vi "Parameter Channel to Strings.vi"(11 "parameter channel definition":T3={"name"="", "default value"=1.0, "unit"="", "parameter definition"={"start index"=0, "size (bits)"=16, "encoding"=enum."BNR", "signed"=TRUE, "multiplier"=1.0, "offset"=0.0}}) -> (3 "parameter channel strings":T1)   [LabVIEW 2020, in "AIM MIL-STD-1553 System Explorer.lvlib" / "Implementation.lvlib" / "Refresh.lvlib"]
uses:
  Refresh.lvlib
  Shared/Parameter Definition.ctl
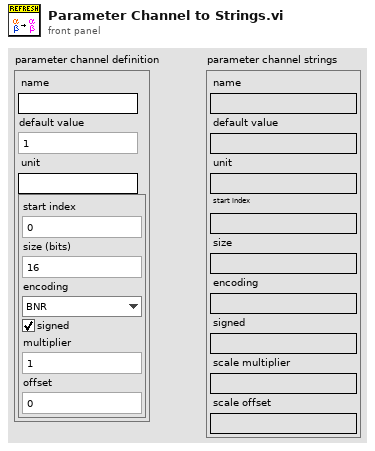
[diagram p1: front panel]
types:
  T1 = cluster{"name":string, "default value":string, "unit":string, "start index":string, "size":string, "encoding":string, "signed":string, "scale multiplier":string, "scale offset":string}
  T2 = typedef "Parameter Definition.ctl" = cluster{"start index":i32, "size (bits)":i32, "encoding":enum16{"BNR", "BCD", "Discrete"}, "signed":bool, "multiplier":dbl, "offset":dbl}
  T3 = cluster{"name":string, "default value":dbl, "unit":string, "parameter definition":T2}
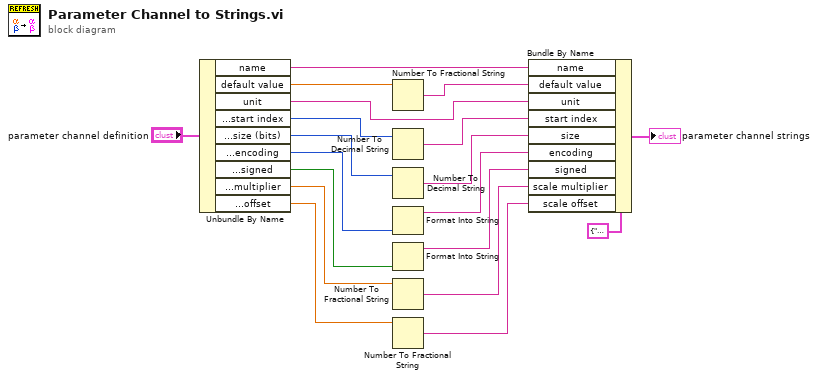
[diagram p0: block diagram]
diagram:
  n1 = Unbundle By Name("parameter channel definition") -> ("name"=w19:string, "default value"=w18:dbl, "unit"=w16:string, "parameter definition.start index"=w15:i32, "parameter definition.size (bits)"=w14:i32, "parameter definition.encoding"=w11:enum16{"BNR", "BCD", "Discrete"}, "parameter definition.signed"=w4:bool, "parameter definition.multiplier"=w10:dbl, "parameter definition.offset"=w9:dbl)
  n2 = Number To Fractional String(number=w18) -> (F-format string=w17:string)  [unwired: 3 in]
  n3 = Number To Decimal String(number=w15) -> (decimal integer string=w13:string)  [unwired: 1 in]
  n4 = Number To Decimal String(number=w14) -> (decimal integer string=w12:string)  [unwired: 1 in]
  n5 = Format Into String(w11) -> (resulting string=w6:string)  [unwired: 3 in, 1 out]
  n6 = Format Into String(w4) -> (resulting string=w5:string)  [unwired: 3 in, 1 out]
  n7 = Number To Fractional String(number=w10) -> (F-format string=w8:string)  [unwired: 3 in]
  n8 = Number To Fractional String(number=w9) -> (F-format string=w7:string)  [unwired: 3 in]
  n9 = Bundle By Name(cluster=T1 {"name"="", "default value"="", "unit"="", "start index"="", "size"="", "encoding"="", "signed"="", "scale multiplier"="", "scale offset"=""} ("parameter channel strings"), "name"=w19, "default value"=w17, "unit"=w16, "start index"=w13, "size"=w12, "encoding"=w6, "signed"=w5, "scale multiplier"=w8, "scale offset"=w7) -> (→"parameter channel strings":T1)
